vi "IncreaseIndexCA.vi"(11 "CA":T1(array[cluster])) -> (3 "updatedCA":T1(array[cluster]))   [LabVIEW 2020]
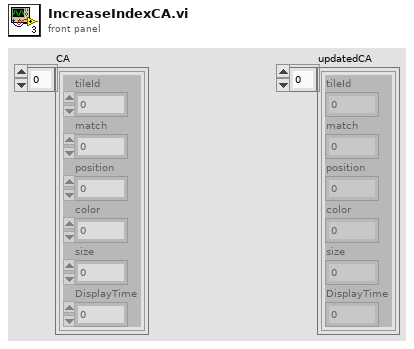
[diagram p1: front panel]
types:
  T1 = cluster{"tileId":i32, "match":i32, "position":i32, "color":u32, "size":i32, "DisplayTime":i32}[]
  T2 = cluster{"tileId":i32, "match":i32, "position":i32, "color":u32, "size":i32, "DisplayTime":i32}
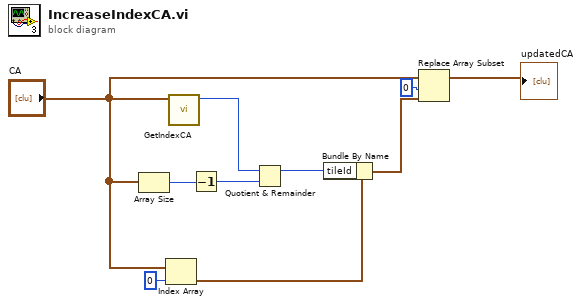
[diagram p0: block diagram]
diagram:
  n1 = Array Size(array="CA") -> (size(s)=w5:i32)
  n2 = Index Array(array="CA", index=0) -> (element=w9:T2)
  n3 = call "GetIndexCA.vi"("CA"="CA") -> ("Current index"=w3:u8)  [unwired: 9 in, 1 out]
  n4 = Decrement(x=w5) -> (x-1=w4:i32)
  n5 = Quotient & Remainder(x=w3, y=w4) -> (x-y*floor(x/y)=w2:i32)  [unwired: 1 out]
  n6 = Bundle By Name(cluster=w9, "tileId"=w2) -> (w7:T2)
  n7 = Replace Array Subset(array="CA", new element=w7, index=0) -> (→"updatedCA":T1)
